vi "Sensor_data_to_value_step1_resolve_sign.vi"(10 "Sensor data":u16, 11 "Sensor type":u8 format="%x") -> (2 "Sensor data resolved sign":i32, 3 "Sensor type out":u8 format="%x")   [LabVIEW 2013]
doc: "Converts raw sensor type data to signed or usigned format. \nADC readings are signed, other usually not.\nDetermines if sensor raw data are signed or unsigned. Output sensor data int32 will give correct result.\n\nUse Sensor_data_to_value_step2_convert for conversion. This function require resolved sign (this VI output)"
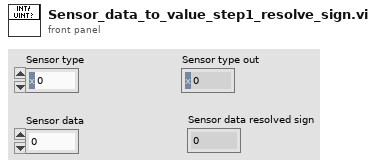
[diagram p1: front panel]
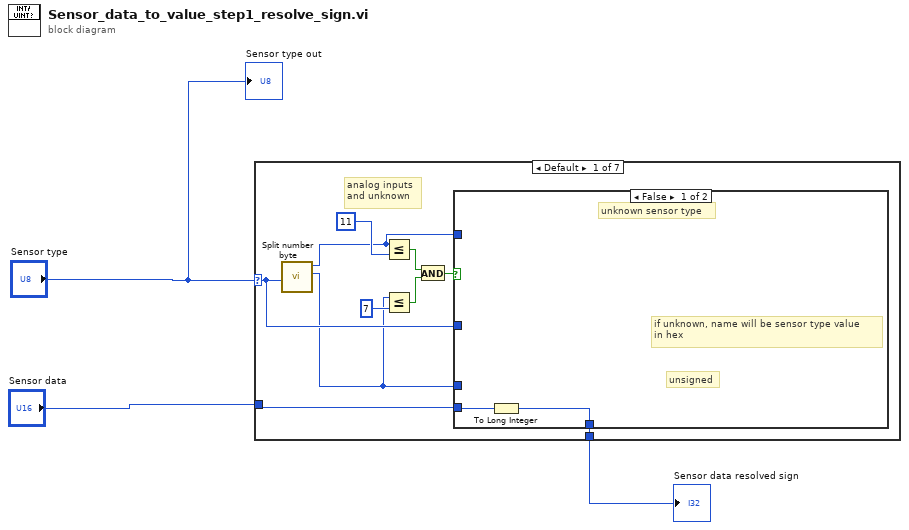
[diagram p0: block diagram]
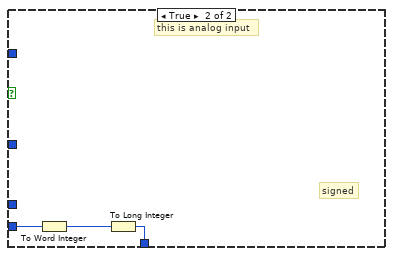
[diagram p2: hidden frame]
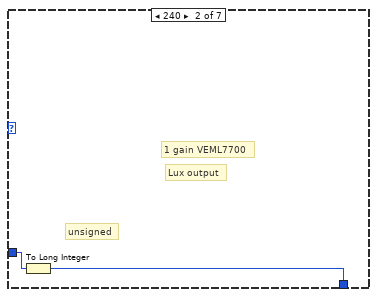
[diagram p3: hidden frame]
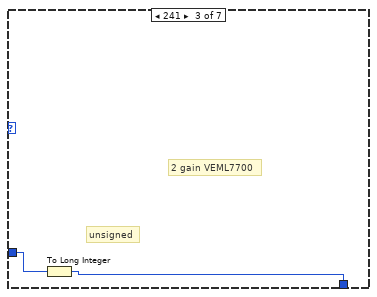
[diagram p4: hidden frame]
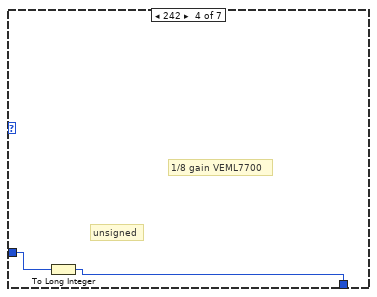
[diagram p5: hidden frame]
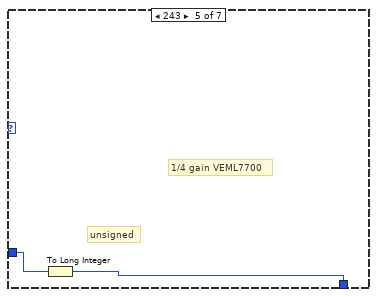
[diagram p6: hidden frame]
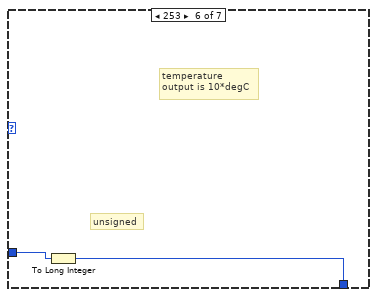
[diagram p7: hidden frame]
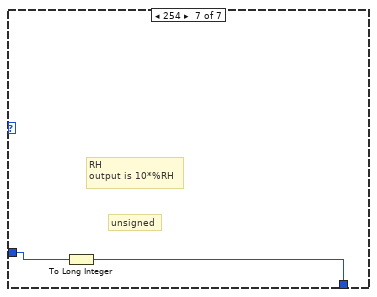
[diagram p8: hidden frame]
diagram:
  n1 = case shown="Default" "Sensor type" {
    selector: "Sensor type" -> [w8 _ _ _ _ _ _]
    tunnel: [w5 w20 w22 w24 w26 w28 w30] -> w1
    tunnel: "Sensor data" -> [w4 w19 w21 w23 w25 w27 w29]
    frame Default {
      # "analog inputs\nand unknown"
      n2 = call "Split number byte.vi"("x"=w8) -> ("lo(x)"=w7:u8, "hi(x)"=w6:u8)  [unwired: 9 in]
      n3 = Less Or Equal?(x=w6, y=u8 11) -> (x <= y?=w11:bool)
      n4 = Less Or Equal?(x=w7, y=u8 7) -> (x <= y?=w10:bool)
      n5 = And(x=w11, y=w10) -> (x .and. y?=w9:bool)
      n6 = case shown="False" w9 {
        tunnel: w7 -> [_ _]
        tunnel: w8 -> [_ _]
        tunnel: w6 -> [_ _]
        tunnel: [w15 w18] -> w5
        tunnel: w4 -> [w14 w16]
        frame False {
          # "unsigned"
          # "if unknown, name will be sensor type value\nin hex"
          # "unknown sensor type"
          n7 = To Long Integer(number=w14) -> (32bit integer=w15:i32)
        }
        frame True {
          # "signed"
          # "this is analog input"
          n8 = To Word Integer(number=w16) -> (16bit integer=w17:i16)
          n9 = To Long Integer(number=w17) -> (32bit integer=w18:i32)
        }
      }
    }
    frame 240 {
      # "unsigned"
      # "Lux output"
      # "1 gain VEML7700"
      n10 = To Long Integer(number=w19) -> (32bit integer=w20:i32)
    }
    frame 241 {
      # "unsigned"
      # "2 gain VEML7700"
      n11 = To Long Integer(number=w21) -> (32bit integer=w22:i32)
    }
    frame 242 {
      # "unsigned"
      # "1/8 gain VEML7700"
      n12 = To Long Integer(number=w23) -> (32bit integer=w24:i32)
    }
    frame 243 {
      # "unsigned"
      # "1/4 gain VEML7700"
      n13 = To Long Integer(number=w25) -> (32bit integer=w26:i32)
    }
    frame 253 {
      # "unsigned"
      # "temperature\noutput is 10*degC"
      n14 = To Long Integer(number=w27) -> (32bit integer=w28:i32)
    }
    frame 254 {
      # "unsigned"
      # "RH\noutput is 10*%RH"
      n15 = To Long Integer(number=w29) -> (32bit integer=w30:i32)
    }
  }
  "Sensor data resolved sign" <- w1
  "Sensor type out" <- "Sensor type"
